vi "fg_queue.vi"(7 "command":T1=enum."read", 8 "error in (no error)":errorcluster, 11 "queue in":refnum<queue>) -> (0 "error out":errorcluster, 3 "queue out":refnum<queue>)   [LabVIEW 2015, in "example_02.lvlib"]
uses:
  example_02.lvlib
  _controls/fg_command.ctl
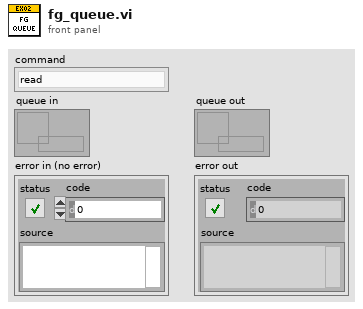
[diagram p1: front panel]
types:
  T1 = typedef "example_02.lvlib/fg_command.ctl" = enum16{"<fg_command>", "initialize", "read", "write", "shutdown"}
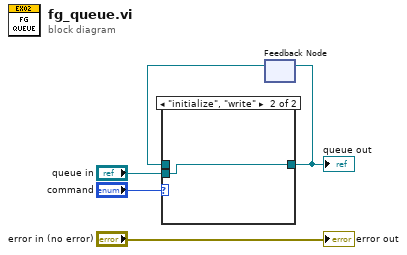
[diagram p0: block diagram]
diagram:
  n1 = feedback #1() -> (w4:refnum<queue>)  [unwired: 1 in]
  n2 = case shown="\"initialize\", \"write\"" "command" {
    tunnel: [w6 w7] -> w5
    tunnel: w4 -> [w6 _]
    tunnel: "queue in" -> [_ w7]
    frame Default {
    }
    frame "initialize", "write" {
    }
  }
  "queue out" <- w5
  n3 = feedback-in #1(w5) -> ()
  "error out" <- "error in (no error)"
